vi "SpatialStart.vi"(0 "Device Info":T1={"Serial Number"=-1, "Channel"=0, "Port"=0}, 1 "Data Interval":i32=-1, 11 "error in (no error)":errorcluster, 12 "Connection":u16(ring) items=["No Preference", "Remote", "Local"], 13 "Timeout (mSec)":i32=5000) -> (4 "Phidget ID":u64, 6 "Serial Number Return":i32, 10 "Attached?":bool, 15 "error out":errorcluster)   [LabVIEW 2020, in "Phidget Spatial.lvlib"]
doc: "${Spatial:StartHeader}"
uses:
  <instrlib>/Phidgets/Phidget Spatial/Phidget Spatial.lvlib
  <instrlib>/Phidgets/Phidget Common/Phidget Common.lvlib
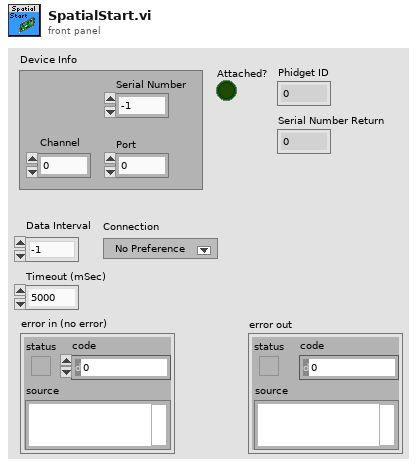
[diagram p1: front panel]
types:
  T1 = cluster{"Serial Number":i32, "Channel":i32, "Port":i32}
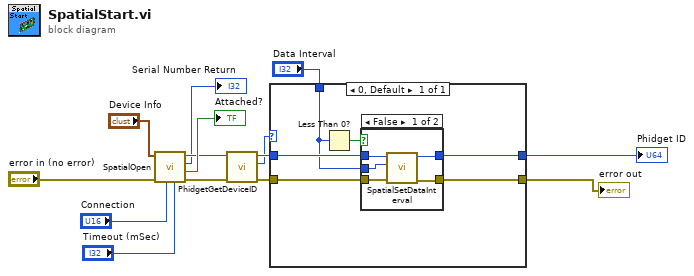
[diagram p0: block diagram]
diagram:
  n1 = call <instrlib>:"SpatialOpen.vi"("Timeout (mSec)"="Timeout (mSec)", "Connection"="Connection", "error in"="error in (no error)", "Device Info"="Device Info") -> ("error out"=w12:errorcluster, "Attached?"=→"Attached?":bool, "Serial Number Return"=→"Serial Number Return":i32, "Phidget ID"=w11:u64)  [unwired: 4 in]
  n2 = call <instrlib>:"PhidgetGetDeviceID.vi"("error in (no error)"=w12, "Device In"=w11) -> ("error out"=w9:errorcluster, "Devie IDs"=w8:u32, "Device Out"=w10:u64)  [unwired: 6 in]
  n3 = case shown="0, Default" w8 {
    tunnel: w9 -> [w19]
    tunnel: [w15] -> w3
    tunnel: w10 -> [w18]
    tunnel: [w16] -> w4
    tunnel: "Data Interval" -> [w17]
    frame 0, Default {
      n4 = Less Than 0?(x=w17) -> (x < 0?=w20:bool)
      n5 = case shown="False" w20 {
        tunnel: w18 -> [w24 w27]
        tunnel: w19 -> [w23 w26]
        tunnel: [w21 w27] -> w16
        tunnel: [w22 w26] -> w15
        tunnel: w17 -> [w25 _]
        frame False {
          n6 = call <instrlib>:"SpatialSetDataInterval.vi"("error in (no error)"=w23, "Interval"=w25, "Device In"=w24) -> ("error out"=w22:errorcluster, "Device Out"=w21:u64)  [unwired: 6 in]
        }
        frame True {
        }
      }
    }
  }
  "error out" <- w3
  "Phidget ID" <- w4
